vi "UpdtCamTestCntrlEvnts.vi"(8 "error in (no error)":errorcluster, 10 "CameraTestingEvnt":T1, 11 "ICameraTestingUI in":refnum<class "ICameraTestingUI.lvclass">) -> (0 "error out":errorcluster, 3 "ICameraTestingUI out":refnum<class "ICameraTestingUI.lvclass">)   [LabVIEW 2020, in "ICameraTestingUI.lvlib" / "ICameraTestingUI.lvclass"]
uses:
  ICameraTestingUI.lvclass
  Camera/ICamera/ICamera/TypeDef/SnapInfo.ctl
  Camera/ICamera/ICamera/ICamera.lvclass
  ICameraTesting/ICameraTesting/TypeDef/FrameRateValReceived.ctl
  ICameraTesting/ICameraTesting/ICameraTesting.lvclass
  ICameraTesting/ICameraTesting/TypeDef/ImgTypeValReceived.ctl
  ICameraTesting/ICameraTesting/TypeDef/ResolutionValReceived.ctl
  Camera/ICamera/ICamera/TypeDef/VideoOptionsCodes.ctl
  ICameraTesting/ICameraTesting/TypeDef/VideoOptCodesReceived.ctl
  ICameraTesting/ICameraTesting/TypeDef/StatusLogUpdate.ctl
  ICameraTesting/ICameraTesting/TypeDef/Events.ctl
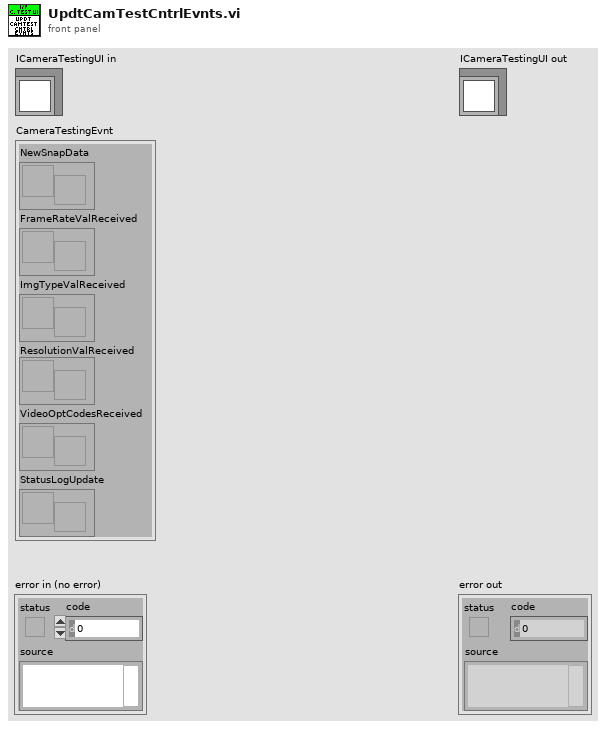
[diagram p1: front panel]
types:
  T1 = typedef "ICameraTesting.lvlib/ICameraTesting.lvclass/Events.ctl" = cluster{"NewSnapData":refnum<user-event>, "FrameRateValReceived":T2, "ImgTypeValReceived":T3, "ResolutionValReceived":T4, "VideoOptCodesReceived":T5, "StatusLogUpdate":T6}
  T2 = typedef "ICameraTesting.lvlib/ICameraTesting.lvclass/FrameRateValReceived.ctl" = refnum<user-event>
  T3 = typedef "ICameraTesting.lvlib/ICameraTesting.lvclass/ImgTypeValReceived.ctl" = refnum<user-event>
  T4 = typedef "ICameraTesting.lvlib/ICameraTesting.lvclass/ResolutionValReceived.ctl" = refnum<user-event>
  T5 = typedef "ICameraTesting.lvlib/ICameraTesting.lvclass/VideoOptCodesReceived.ctl" = refnum<user-event>
  T6 = typedef "ICameraTesting.lvlib/ICameraTesting.lvclass/StatusLogUpdate.ctl" = refnum<user-event>
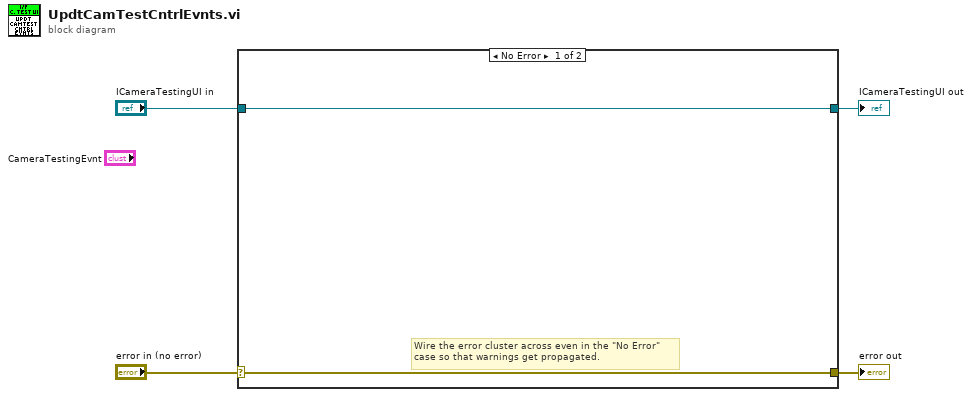
[diagram p0: block diagram]
diagram:
  n1 = case shown="No Error" "error in (no error)" {
    selector: "error in (no error)" -> [w5 w8]
    tunnel: [w5 w8] -> w3
    tunnel: [w6 w7] -> w1
    tunnel: "ICameraTestingUI in" -> [w6 w7]
    frame No Error {
      # "Wire the error cluster across even in the \"No Error\"\ncase so that warnings get propagated."
    }
    frame Error {
    }
  }
  "error out" <- w3
  "ICameraTestingUI out" <- w1
